vi "Controller Queue Handler.vi"(7 "Action":T3, 8 "error in (no error)":errorcluster, 10 "Message in":T1={"Message Info"=enum."Initial", "Message Data"=variant}, 11 "Queue in":refnum<queue>) -> (0 "error out":errorcluster, 2 "Message out":T1={"Message Info"=enum."Initial", "Message Data"=variant}, 3 "Queue out":refnum<queue>)   [LabVIEW 2017]
uses:
  Type Definitions/Queue FG Options.ctl
  Type Definitions/Controller Message.ctl
  Type Definitions/Controller States.ctl
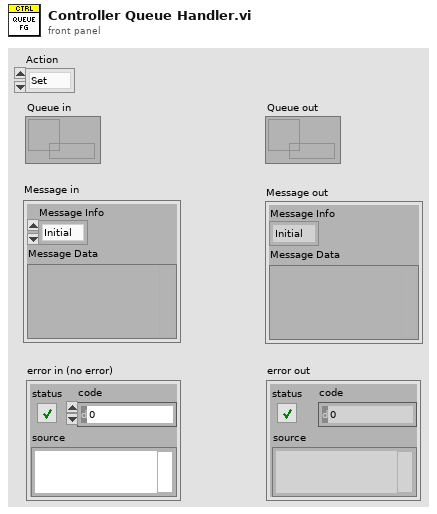
[diagram p1: front panel]
types:
  T1 = typedef "Controller Message.ctl" = cluster{"Message Info":T2, "Message Data":variant}
  T2 = typedef "Controller States.ctl" = enum16{"Timeout", "Initial", "Login", "Idle", "Balance Inquiry", "Deposit", "Withdrawal", "Fast Cash", "Terminate", "Wait on Exit", "Shutdown", "Error Handler"}
  T3 = typedef "Queue FG Options.ctl" = enum16{"Set", "Get", "Read", "Write", "Destroy"}
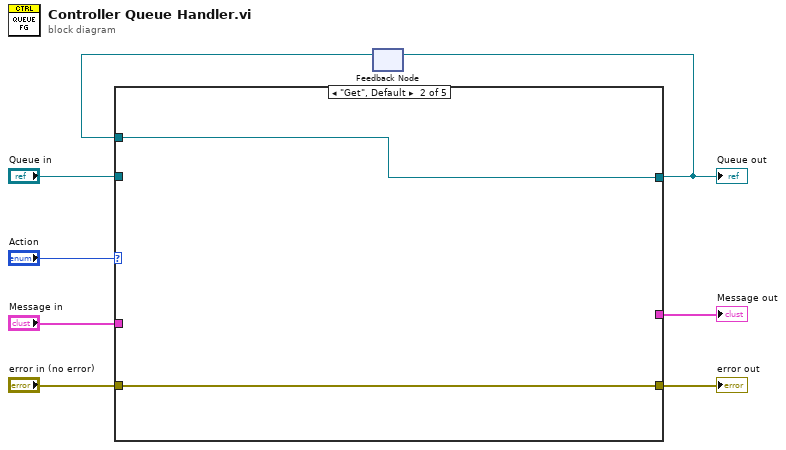
[diagram p0: block diagram]
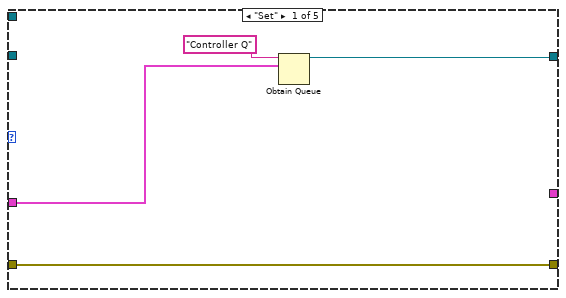
[diagram p2: hidden frame]
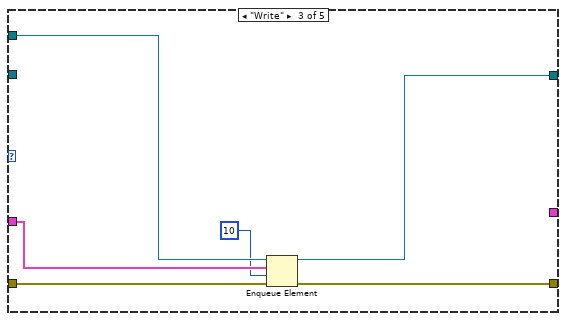
[diagram p3: hidden frame]
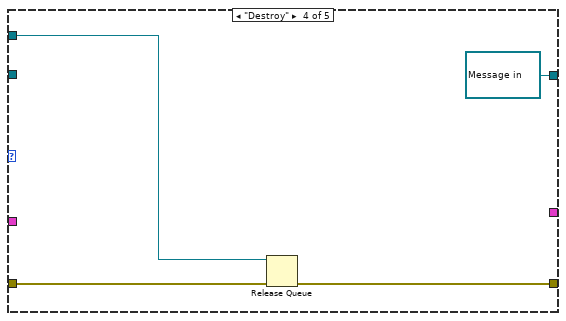
[diagram p4: hidden frame]
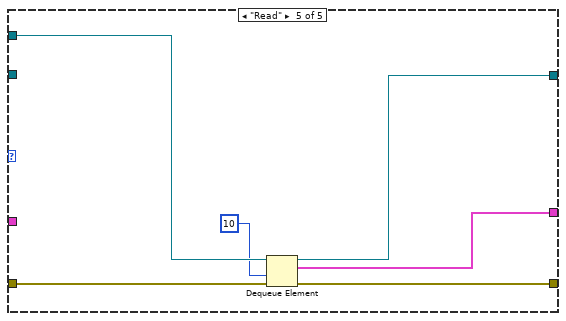
[diagram p5: hidden frame]
diagram:
  n1 = feedback #1() -> (w5:refnum<queue>)  [unwired: 1 in]
  n2 = case shown="\"Get\", Default" "Action" {
    tunnel: "error in (no error)" -> [w12 w14 w20 w24 w30]
    tunnel: [w12 w14 w19 w23 w29] -> w6
    tunnel: w5 -> [_ w13 w18 w22 w26]
    tunnel: "Message in" -> [w10 _ w16 _ _]
    tunnel: [_ _ _ _ w28] -> w3
    tunnel: [w11 w13 w17 refnum<queue> refnum ("queue out") w27] -> w1
    tunnel: "Queue in" -> [_ _ _ _ _]
    frame "Set" {
      n3 = Obtain Queue(name (unnamed)="Controller Q", element data type=w10) -> (queue out=w11:refnum<queue>)  [unwired: 3 in, 2 out]
    }
    frame "Get", Default {
    }
    frame "Write" {
      n4 = Enqueue Element(queue=w18, element=w16, timeout in ms (-1)=10, error in (no error)=w20) -> (queue out=w17:refnum<queue>, error out=w19:errorcluster)  [unwired: 1 out]
    }
    frame "Destroy" {
      n5 = Release Queue(queue=w22, error in (no error)=w24) -> (error out=w23:errorcluster)  [unwired: 1 in, 2 out]
    }
    frame "Read" {
      n6 = Dequeue Element(queue=w26, timeout in ms (-1)=10, error in (no error)=w30) -> (queue out=w27:refnum<queue>, element=w28:T1, error out=w29:errorcluster)  [unwired: 1 out]
    }
  }
  "error out" <- w6
  "Message out" <- w3
  "Queue out" <- w1
  n7 = feedback-in #1(w1) -> ()
